vi "CharToASCII.vi"(1 "Character":string) -> (0 "ASCII Code":u8)   [LabVIEW 2011]
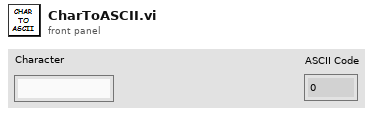
[diagram p1: front panel]
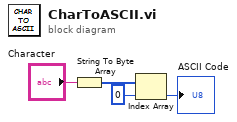
[diagram p0: block diagram]
diagram:
  n1 = String To Byte Array(string="Character") -> (unsigned byte array=w3:u8[])
  n2 = Index Array(array=w3, index=0 ("索引")) -> (element=→"ASCII Code":u8)
